vi "MutationHistoryToTable.vi"(8 "error in (no error)":errorcluster, 11 "Mutation History":T1 {"LabVIEW Version" format="%.0x"}) -> (2 "Class Default Data":variant[](array[variant]), 3 "Table":string[][](array[string]))   [LabVIEW 2019, in "MutationHistoryGUI.lvlib"]
uses:
  MutationHistoryGUI.lvlib
  <vilib>/Utility/EditLVLibs/LVClass/Mutation History.ctl
  <vilib>/Utility/EditLVLibs/LVClass/Mutation Record.ctl
  <vilib>/Utility/EditLVLibs/LibVersion.ctl
  <resource>/Framework/Providers/BlueSerializationProviderShared/BlueSerializationProviderShared.lvlib
  <vilib>/Utility/EditLVLibs/Edit LVLibs.lvlib
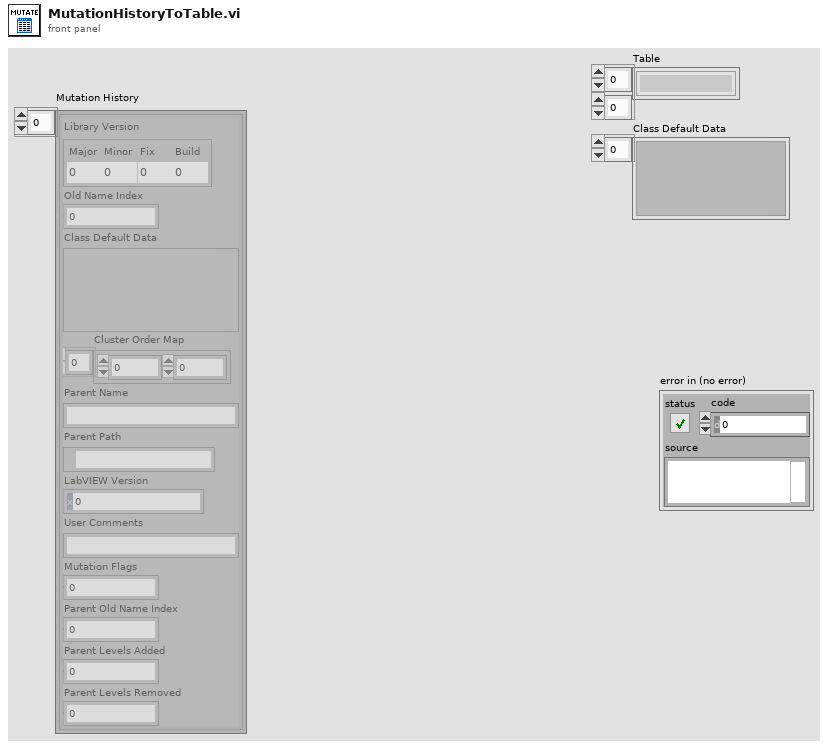
[diagram p1: front panel]
types:
  T1 = typedef "Edit LVLibs.lvlib/Mutation History.ctl" = T2[]
  T2 = typedef "Edit LVLibs.lvlib/Mutation Record.ctl" = cluster{"Library Version":T3, "Old Name Index":u8, "Class Default Data":variant, "Cluster Order Map":u32[], "Parent Name":string, "Parent Path":path, "LabVIEW Version":u32, "User Comments":string, "Mutation Flags":u8, "Parent Old Name Index":u8, "Parent Levels Added":u16, "Parent Levels Removed":u16}
  T3 = typedef "Edit LVLibs.lvlib/LibVersion.ctl" = cluster{"Major":u16, "Minor":u16, "Fix":u16, "Build":u16}
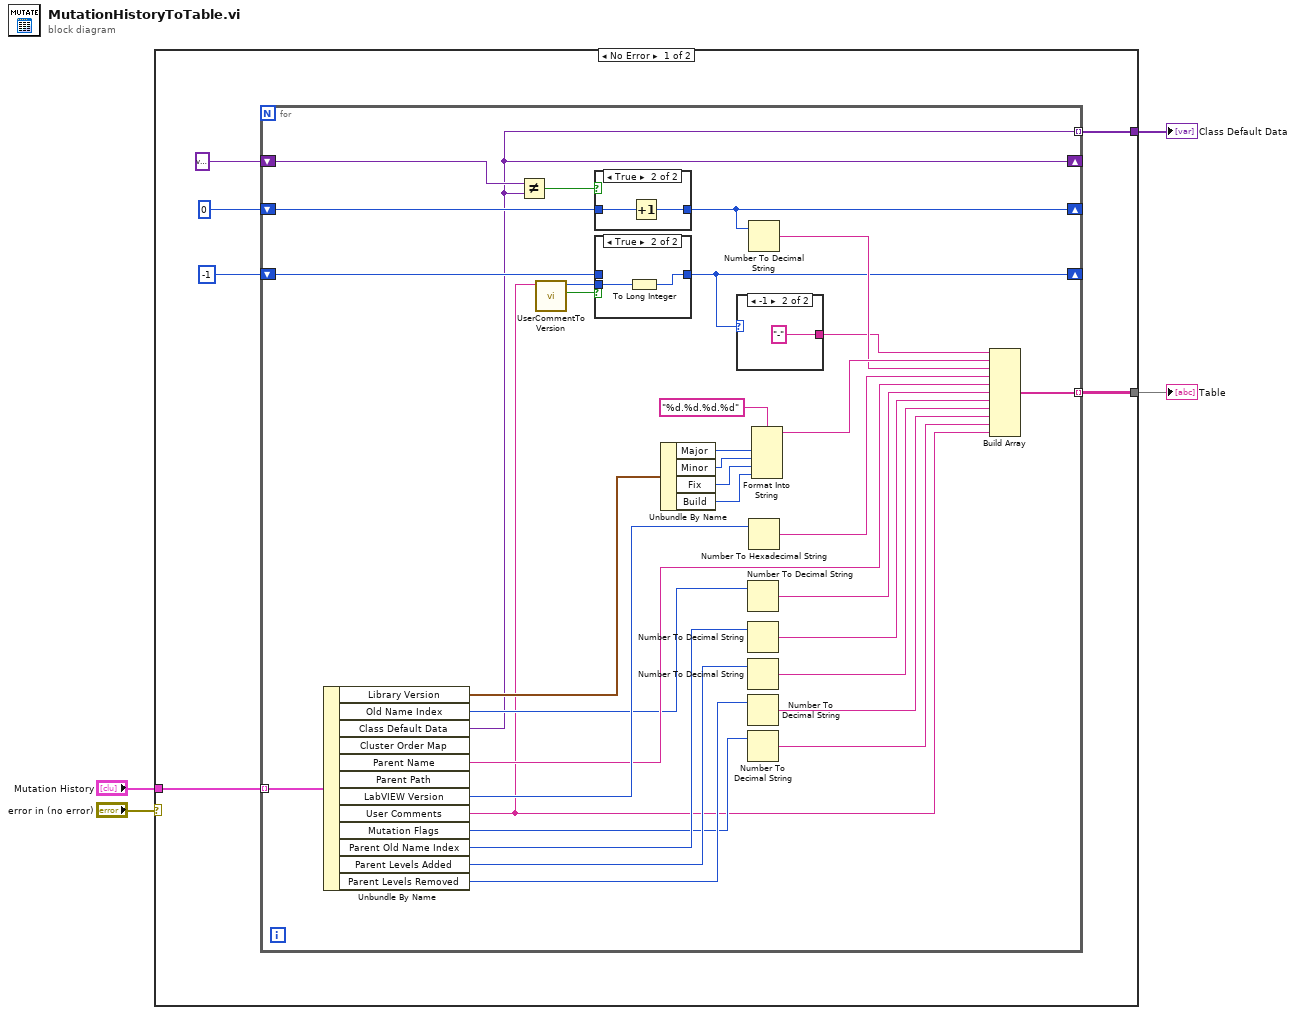
[diagram p0: block diagram]
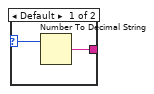
[diagram p3: hidden frame]
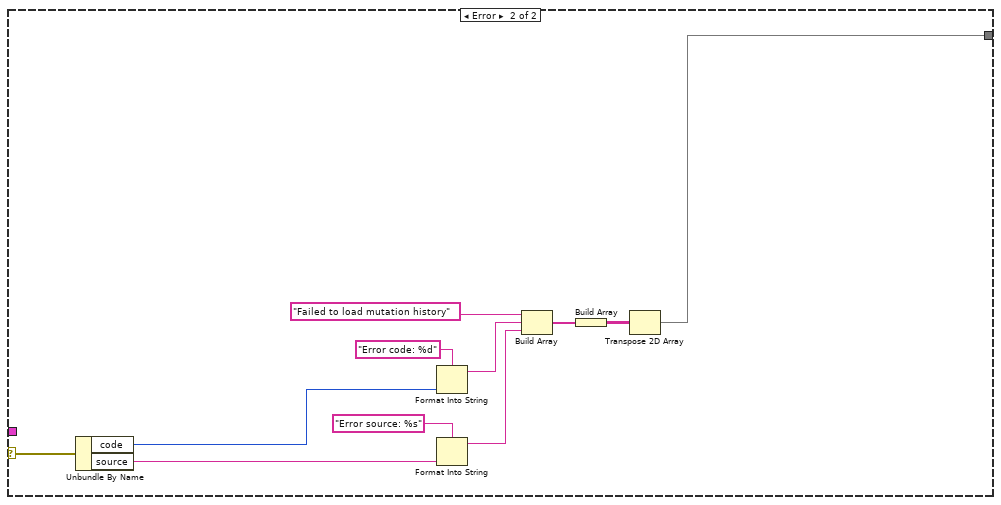
[diagram p5: hidden frame]
diagram:
  n1 = case shown="No Error" "error in (no error)" {
    selector: "error in (no error)" -> [_ w64]
    tunnel: "Mutation History" -> [w10 _]
    tunnel: [w6 w54] -> w3
    tunnel: [w5 _] -> w2
    frame No Error {
      n2 = for {
        tunnel: w10 -> [w44] mode=indexing
        shift-right: [w11] -> _
        shift-left: variant -> [w36]
        shift-right: [w33] -> _
        shift-left: 0 -> [w34]
        tunnel: [w17] -> w6 mode=indexing
        shift-right: [w13] -> _
        shift-left: -1 -> [w15]
        tunnel: [w11] -> w5 mode=indexing
        n3 = Unbundle By Name(w44) -> ("Library Version"=w42:T3, "Old Name Index"=w27:u8, "Class Default Data"=w11:variant, "Parent Name"=w29:string, "LabVIEW Version"=w31:u32, "User Comments"=w18:string, "Mutation Flags"=w20:u8, "Parent Old Name Index"=w26:u8, "Parent Levels Added"=w24:u16, "Parent Levels Removed"=w22:u16)  [unwired: 2 out]
        n4 = Not Equal?(x=w36, y=w11) -> (x != y?=w35:bool)
        n5 = call <resource>:"UserCommentToVersion.vi"("User Comment"=w18) -> ("BlueSerializableVersion found?"=w16:bool, "BlueSerializableVersion"=w14:u16)  [unwired: 9 in]
        n6 = case shown="True" w35 {
          tunnel: w34 -> [w45 w47]
          tunnel: [w45 w46] -> w33
          frame False {
          }
          frame True {
            n7 = Increment(x=w47) -> (x+1=w46:i32)
          }
        }
        n8 = case shown="True" w16 {
          tunnel: w15 -> [w51 _]
          tunnel: [w51 w52] -> w13
          tunnel: w14 -> [_ w53]
          frame False {
          }
          frame True {
            n9 = To Long Integer(number=w53) -> (32bit integer=w52:i32)
          }
        }
        n10 = Unbundle By Name(w42) -> ("Major"=w41:u16, "Minor"=w40:u16, "Fix"=w39:u16, "Build"=w38:u16)
        n11 = case shown="-1" w13 {
          selector: w13 -> [w49 _]
          tunnel: [w48 "-"] -> w12
          frame Default {
            n12 = Number To Decimal String(number=w49) -> (decimal integer string=w48:string)  [unwired: 1 in]
          }
          frame -1 {
          }
        }
        n13 = Number To Decimal String(number=w27) -> (decimal integer string=w28:string)  [unwired: 1 in]
        n14 = Number To Decimal String(number=w26) -> (decimal integer string=w25:string)  [unwired: 1 in]
        n15 = Number To Decimal String(number=w24) -> (decimal integer string=w23:string)  [unwired: 1 in]
        n16 = Number To Decimal String(number=w22) -> (decimal integer string=w21:string)  [unwired: 1 in]
        n17 = Number To Decimal String(number=w20) -> (decimal integer string=w19:string)  [unwired: 1 in]
        n18 = Number To Decimal String(number=w33) -> (decimal integer string=w32:string)  [unwired: 1 in]
        n19 = Number To Hexadecimal String(2:w31) -> (0:w30:string)  [unwired: 1 in]
        n20 = Format Into String(format string="%d.%d.%d.%d", w41, w40, w39, w38) -> (resulting string=w37:string)  [unwired: 2 in, 1 out]
        n21 = Build Array(w12, w37, w32, w30, w29, w28, w25, w23, w21, w19, w18) -> (w17:string[])
      }
    }
    frame Error {
      n22 = Unbundle By Name(w64) -> ("code"=w61:i32, "source"=w60:string)
      n23 = Format Into String(format string="Error code: %d", w61) -> (resulting string=w58:string)  [unwired: 2 in, 1 out]
      n24 = Format Into String(format string="Error source: %s", w60) -> (resulting string=w57:string)  [unwired: 2 in, 1 out]
      n25 = Build Array("Failed to load mutation history", w58, w57) -> (w56:string[])
      n26 = Build Array(w56) -> (w55:string[][])
      n27 = Transpose 2D Array(2D array=w55) -> (transposed array=w54:string[][])
    }
  }
  "Table" <- w3
  "Class Default Data" <- w2
